vi "UDP Data Link - Configuration Utilities - Get Local IP Address State.vi"(8 "error in (no error)":errorcluster, 11 "Item Ref in":T1 format="%.0x") -> (0 "error out":errorcluster, 2 "State":T2(ring), 3 "Item Ref out":T1 format="%.0x")   [LabVIEW 2012, in "UDP Data Link System Explorer.lvlib"]
doc: "Set the <b>IP Address of Local NIC</b> disabled state."
uses:
  UDP Data Link System Explorer.lvlib
  <vilib>/NI Veristand/Custom Device API/Custom Device Item Ref.ctl
  Shared/UDP Data Link Global.vi
  <vilib>/NI Veristand/Custom Device API/Get Item Property (Variant).vi
  <vilib>/NI Veristand/Custom Device API/Custom Device API.lvlib
  Shared/UDP Data Link Shared.lvlib
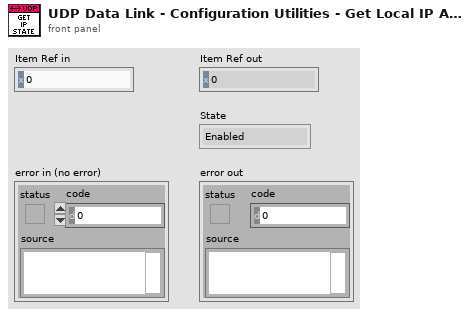
[diagram p1: front panel]
types:
  T1 = typedef "Custom Device API.lvlib/Custom Device Item Ref.ctl" = u64
  T2 = enum8{"Enabled", "Disabled", "Disabled and Grayed Out"}
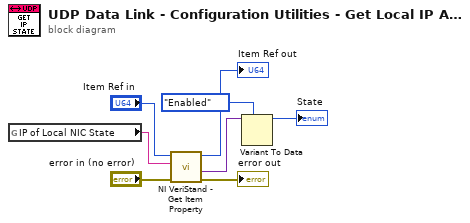
[diagram p0: block diagram]
diagram:
  n1 = global read "UDP Data Link Global.vi" "IP of Local NIC State"() -> (w6:string)
  n2 = call-poly <vilib>:"NI VeriStand - Get Item Property.vi"("error in (no error)"="error in (no error)", "Property Name"=w6, "Item Ref in"="Item Ref in") -> ("error out"=→"error out":errorcluster, "Value"=w5:variant, "Item Ref out"=→"Item Ref out":T1)  [unwired: 5 in, 1 out]
  n3 = Variant To Data(type=T2."Enabled" ("Disabled"), Variant=w5) -> (data=→"State":T2)  [unwired: 1 in, 1 out]
